vi "ScaleKbyR2.vi"(10 "dx":dbl, 11 "K":dbl[](array[numeric])) -> (3 "Kscaled":dbl[](array[numeric]))   [LabVIEW 2014]
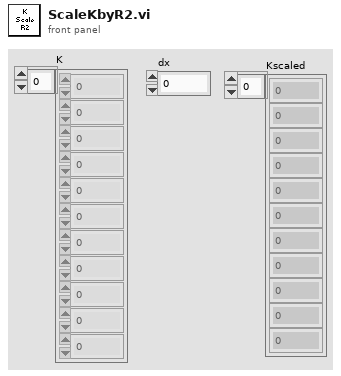
[diagram p1: front panel]
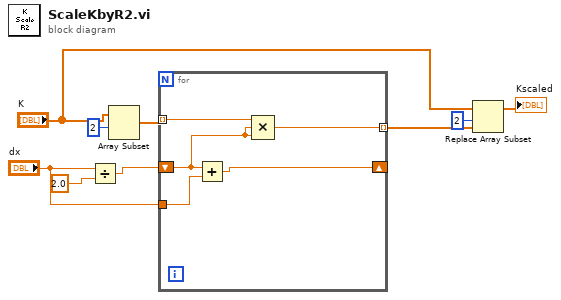
[diagram p0: block diagram]
diagram:
  n1 = Divide(x="dx", y=2.0) -> (x/y=w8:dbl)
  n2 = Array Subset(array="K", index=2) -> (w6:dbl[])  [unwired: 1 in]
  n3 = for {
    tunnel: w6 -> [w12] mode=indexing
    shift-right: [w13] -> _
    shift-left: w8 -> [w11]
    tunnel: "dx" -> [w14]
    tunnel: [w10] -> w3 mode=indexing
    n4 = Add(x=w11, y=w14) -> (x+y=w13:dbl)
    n5 = Compound Arithmetic op=MULTIPLY(w12, w11, w11) -> (w10:dbl)
  }
  n6 = Replace Array Subset(array="K", new element=w3, index=2) -> (→"Kscaled":dbl[])
